vi "Dispose.vi"(8 "error in (no error)":errorcluster, 11 "CameraTestingProxyAPI in":refnum<class "CameraTestingProxyAPI.lvclass">) -> (0 "error out":errorcluster, 3 "CameraTestingProxyAPI out":refnum<class "CameraTestingProxyAPI.lvclass">)   [LabVIEW 2020, in "CameraTestingProxy.lvlib" / "CameraTestingProxyAPI.lvclass"]
uses:
  CameraTestingProxyAPI.lvclass
  CameraTestingProxyAPI.lvclass/CameraTestingProxyAPI.ctl
  0e34f1ae-e0ba-49be-ab8b-7b928111ee75.vi
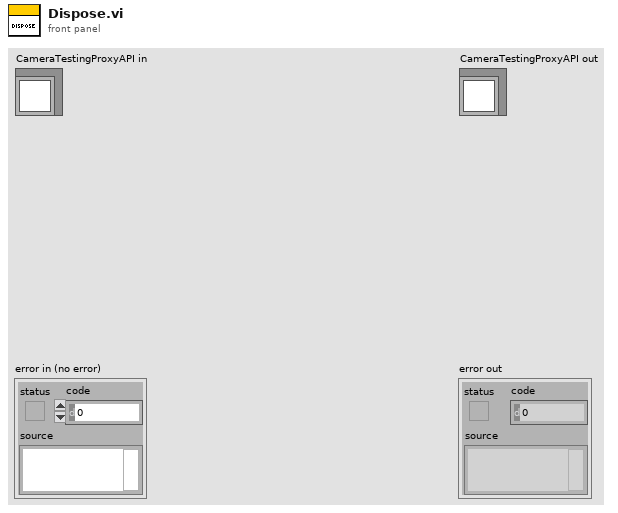
[diagram p1: front panel]
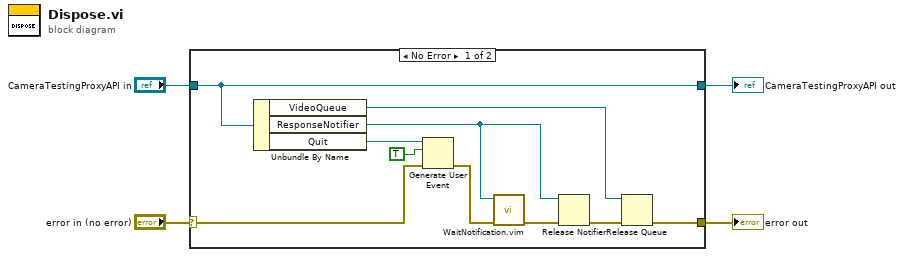
[diagram p0: block diagram]
diagram:
  n1 = case shown="No Error" "error in (no error)" {
    selector: "error in (no error)" -> [w13 w16]
    tunnel: [w9 w16] -> w1
    tunnel: [w10 w15] -> w3
    tunnel: "CameraTestingProxyAPI in" -> [w10 w15]
    frame No Error {
      n2 = Unbundle By Name(w10) -> ("VideoQueue"=w6:refnum<queue>, "ResponseNotifier"=w5:refnum<notifier>, "Quit"=w14:refnum<user-event>)
      n3 = Generate User Event(user event=w14, event data cluster=TRUE ("event data"), error in=w13) -> (error out=w11:errorcluster)  [unwired: 1 in, 1 out]
      n4 = call "WaitNotification.vim"("error in (no error)"=w11, "ResponseNotifier"=w5) -> ("error out"=w8:errorcluster)  [unwired: 8 in, 1 out]
      n5 = Release Notifier(notifier=w5, error in (no error)=w8) -> (error out=w7:errorcluster)  [unwired: 1 in, 2 out]
      n6 = Release Queue(queue=w6, error in (no error)=w7) -> (error out=w9:errorcluster)  [unwired: 1 in, 2 out]
    }
    frame Error {
    }
  }
  "error out" <- w1
  "CameraTestingProxyAPI out" <- w3
